vi "Load Project From Index.vi"(8 "error in (no error)":errorcluster, 10 "Projext Path":path, 11 "LUnit Test Suite in":refnum<class "LUnit Test Suite.lvclass">) -> (0 "error out":errorcluster, 3 "LUnit Test Suite out":refnum<class "LUnit Test Suite.lvclass">)   [LabVIEW 2020, in "Test Finder.lvclass"]
uses:
  Test Finder.lvclass
  API/LUnit Test Suite/LUnit Test Suite.lvclass
  C:/git/astemes-lunit/source/Core/Runnable/Runnable.lvclass
  Test Finder.lvclass/Test Finder.ctl
  C:/git/astemes-lunit/source/API/LUnit Test Suite/LUnit Test Suite.lvclass
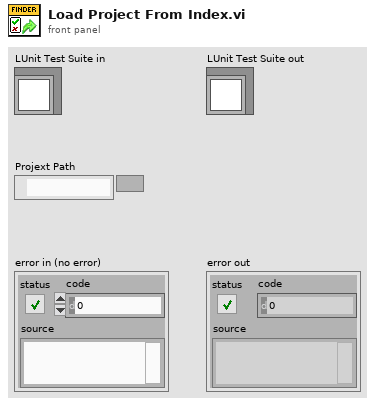
[diagram p1: front panel]
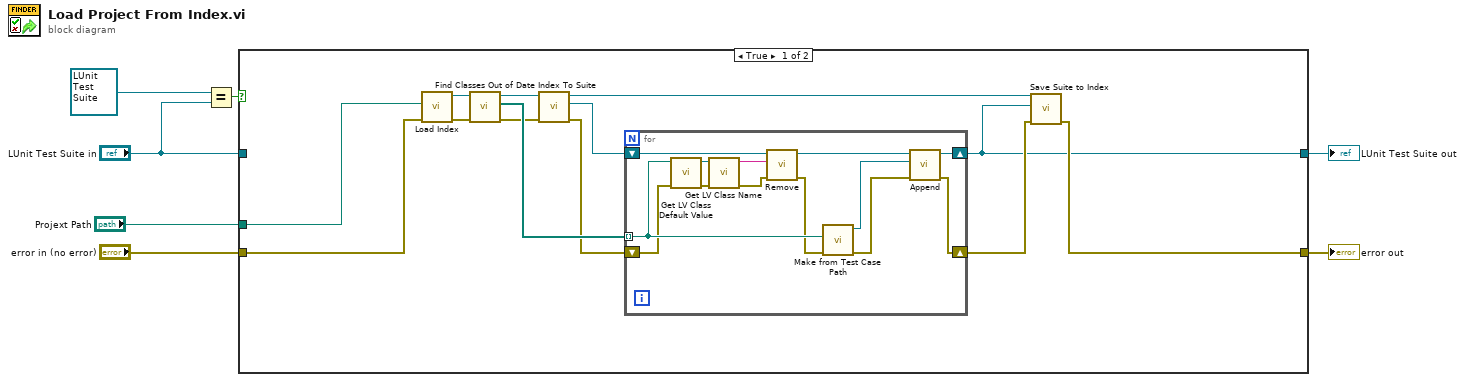
[diagram p0: block diagram]
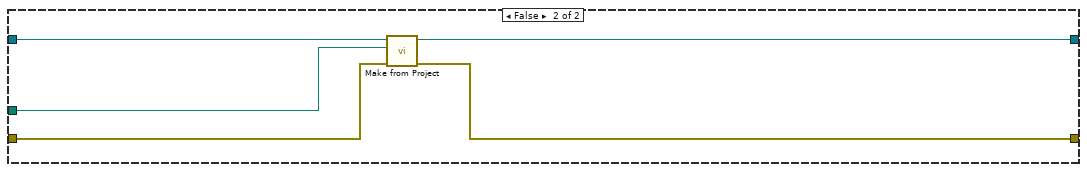
[diagram p2: hidden frame]
diagram:
  n1 = Equal?(x=refnum<class "LUnit Test Suite.lvclass"> refnum ("y"), y="LUnit Test Suite in") -> (x = y?=w2:bool)
  n2 = case shown="True" w2 {
    tunnel: [w8 w38] -> w1
    tunnel: "Projext Path" -> [w20 w37]
    tunnel: "error in (no error)" -> [w16 w36]
    tunnel: [w9 w35] -> w5
    tunnel: "LUnit Test Suite in" -> [_ w34]
    frame True {
      n3 = call "Load Index.vi"("error in (no error)"=w16, "Project Path"=w20) -> ("error out"=w18:errorcluster, "Test Finder out"=w19:refnum<class "Test Finder.lvclass">)  [unwired: 8 in]
      n4 = call "Find Classes Out of Date.vi"("error in (no error)"=w18, "Test Finder In"=w19) -> ("error out"=w14:errorcluster, "Outdated Test Class paths"=w17:path[], "Test Finder Out"=w15:refnum<class "Test Finder.lvclass">)  [unwired: 7 in]
      n5 = call "Index To Suite.vi"("error in (no error)"=w14, "Test Finder In"=w15) -> ("error out"=w13:errorcluster, "Suite"=w12:refnum<class "LUnit Test Suite.lvclass">, "Test Finder Out"=w11:refnum<class "Test Finder.lvclass">)  [unwired: 7 in]
      n6 = for {
        tunnel: w17 -> [w25] mode=indexing
        shift-right: [w32] -> w8
        shift-left: w12 -> [w33]
        shift-right: [w31] -> w10
        shift-left: w13 -> [w23]
        n7 = call <vilib>:"Get LV Class Default Value.vi"("error in (no error)"=w23, "class path"=w25) -> ("error out"=w27:errorcluster, "object"=w26:refnum<class>)  [unwired: 8 in]
        n8 = call <vilib>:"Get LV Class Name.vi"("error in (no error)"=w27, "object"=w26) -> ("error out"=w22:errorcluster, "class name"=w24:string)  [unwired: 8 in]
        n9 = call "Remove.vi"("error in (no error)"=w22, "Test to Remove"=w24, "LUnit Test Suite In"=w33) -> ("error out"=w21:errorcluster, "LUnit Test Suite Out"=w28:refnum<class "LUnit Test Suite.lvclass">)  [unwired: 7 in]
        n10 = call "Make from Test Case Path.vi"("error in (no error)"=w21, "Test Case"=w25) -> ("error out"=w30:errorcluster, "LUnit Test Suite Out"=w29:refnum<class "LUnit Test Suite.lvclass">)  [unwired: 8 in]
        n11 = call "Append.vi"("error in (no error)"=w30, "Runnable"=w29, "LUnit Test Suite In"=w28) -> ("error out"=w31:errorcluster, "LUnit Test Suite Out"=w32:refnum<class "LUnit Test Suite.lvclass">)  [unwired: 7 in]
      }
      n12 = call "Save Suite to Index.vi"("error in (no error)"=w10, "Suite"=w8, "Test Finder In"=w11) -> ("error out"=w9:errorcluster)  [unwired: 8 in]
    }
    frame False {
      n13 = call "Make from Project.vi"("error in (no error)"=w36, "Project Path"=w37, "LUnit Test Suite In"=w34) -> ("error out"=w35:errorcluster, "LUnit Test Suite Out"=w38:refnum<class "LUnit Test Suite.lvclass">)  [unwired: 7 in]
    }
  }
  "LUnit Test Suite out" <- w1
  "error out" <- w5
